vi "Slice Average calc wrapper.vi"(6 "Plot ref":refnum<vi>, 7 "update plot":T2, 10 "HasData?":bool[](array[boolean]), 11 "Plot (unix)":T5[](array[typedef])) -> (3 "Plot (unix)":T5[](array[typedef]), 5 "RightClickCache.slice":T1[](array[typedef]))   [LabVIEW 2021, in "RocketPlot.lvlib"]
uses:
  RocketPlot.lvlib
  TypeDefs/plot datapoint.ctl
  TypeDefs/update plot queue data.ctl
  TypeDefs/RightClickType.ctl
  <vilib>/Utility/miscctls.llb/LVPoint32TypeDef.ctl
  TypeDefs/Slice average.ctl
  b0f39d84-27d9-4b84-b8c3-cf78f35fa78a.vi
  b8f4d68e-665a-4d51-938f-4be5908799fb.vi
  0a7e6c96-3213-4357-8ae2-7647ccf6d38e.vi
  de1cbfd4-f4b0-4655-8da2-e779fdd6673d.vi
  <userlib>/bjustice/Ring Buffer for Time Series Data Strict Accessor/SubVIs/Search for time to keep.vi
  Slice Average calc.vi/aeb3b9b0-3d0b-48fb-8ca9-3c9e8c208765.vi
  Slice Average calc.vi/43998882-4a9d-44ca-a800-b6f182c48d79.vi
  <userlib>/bjustice/Ring Buffer for Time Series Data Strict Accessor/Unix time epoch/Unix_Epoch_in_Labview.vi
  <userlib>/bjustice/Ring Buffer for Time Series Data Strict Accessor/SubVIs/Search for oldest time to keep.vi
  <userlib>/bjustice/Ring Buffer for Time Series Data Strict Accessor/SubVIs/Search for newest time to keep.vi
  <vilib>/Analysis/baseanly.llb/Std Deviation and Variance.vi
  <vilib>/Analysis/8numeric.llb/Uneven Numeric Integration.vi
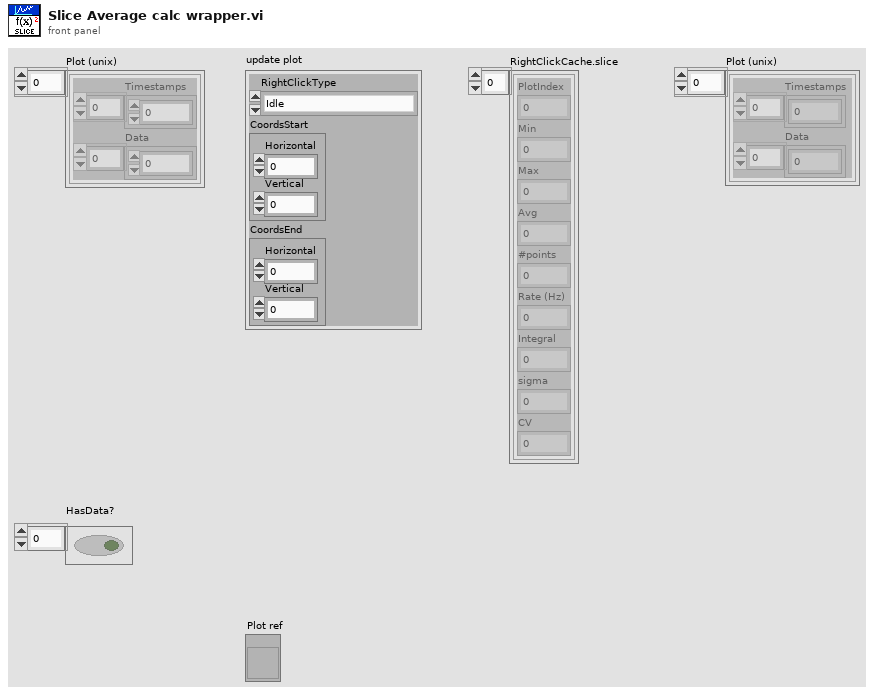
[diagram p1: front panel]
types:
  T1 = typedef "RocketPlot.lvlib/Slice average.ctl" = cluster{"PlotIndex":i32, "Min":dbl, "Max":dbl, "Avg":dbl, "#points":u32, "Rate (Hz)":dbl, "Integral":dbl, "sigma":dbl, "CV":dbl}
  T2 = typedef "RocketPlot.lvlib/update plot queue data.ctl" = cluster{"RightClickType":T3, "CoordsStart":T4, "CoordsEnd":T4}
  T3 = typedef "RocketPlot.lvlib/RightClickType.ctl" = enum16{"Idle", "Delta", "SliceAvg", "Identify"}
  T4 = typedef "LVPoint32TypeDef.ctl" = cluster{"Horizontal":i32, "Vertical":i32}
  T5 = typedef "RocketPlot.lvlib/plot datapoint.ctl" = cluster{"Timestamps":u64[], "Data":dbl[]}
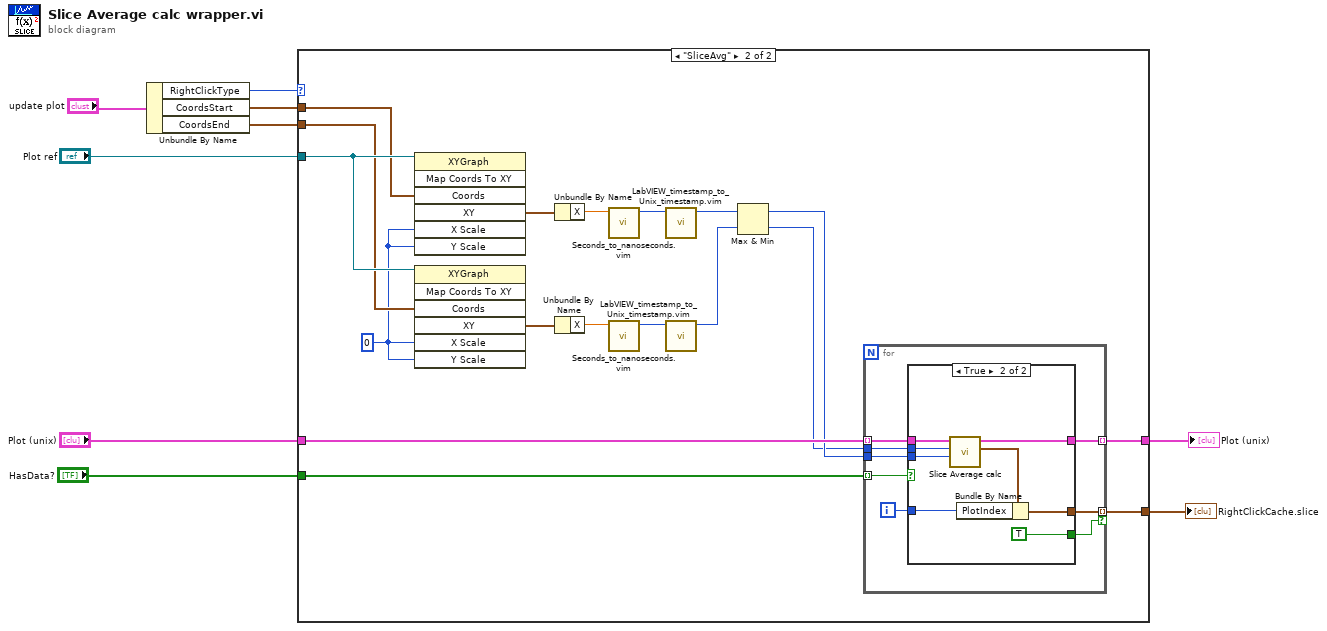
[diagram p0: block diagram]
diagram:
  n1 = Unbundle By Name("update plot") -> ("RightClickType"=w4:T3, "CoordsStart"=w3:T4, "CoordsEnd"=w2:T4)
  n2 = case shown="\"SliceAvg\"" w4 {
    tunnel: "Plot (unix)" -> [w10 w28]
    tunnel: [w10 w27] -> w8
    tunnel: "Plot ref" -> [_ w26]
    tunnel: "HasData?" -> [_ w25]
    tunnel: w3 -> [_ w24]
    tunnel: w2 -> [_ w23]
    tunnel: [_ w22] -> w1
    frame Default {
    }
    frame "SliceAvg" {
      w21 = 0 ("X Scale")
      n3 = invoke class="XYGraph" method="Map Coords To XY"(reference=w26, "Coords"=w24, "X Scale"=w21, "Y Scale"=w21) -> ("XY"=w20:cluster{"X":dbl, "Y":dbl})  [unwired: 3 in, 6 out]
      n4 = invoke class="XYGraph" method="Map Coords To XY"(reference=w26, "Coords"=w23, "X Scale"=w21, "Y Scale"=w21) -> ("XY"=w19:cluster{"X":dbl, "Y":dbl})  [unwired: 3 in, 6 out]
      n5 = Unbundle By Name(w20) -> ("X"=w15:dbl)
      n6 = Unbundle By Name(w19) -> ("X"=w12:dbl)
      n7 = call "Seconds_to_nanoseconds.vim"("timestamp (seconds)"=w15) -> ("timestamp (nanoseconds)"=w16:u64)  [unwired: 10 in]
      n8 = call "Seconds_to_nanoseconds.vim"("timestamp (seconds)"=w12) -> ("timestamp (nanoseconds)"=w13:u64)  [unwired: 10 in]
      n9 = call "LabVIEW_timestamp_to_Unix_timestamp.vim"("LabVIEW timestamp (nanoseconds)"=w16) -> ("Unix timestamp (nanoseconds)"=w14:u64)  [unwired: 10 in]
      n10 = call "LabVIEW_timestamp_to_Unix_timestamp.vim"("LabVIEW timestamp (nanoseconds)"=w13) -> ("Unix timestamp (nanoseconds)"=w11:u64)  [unwired: 10 in]
      n11 = Max & Min(x=w14, y=w11) -> (max(x,y)=w18:u64, min(x,y)=w17:u64)
      n12 = for {
        tunnel: w28 -> [w36] mode=indexing
        tunnel: [w35] -> w27 mode=indexing
        tunnel: [w34] -> w22 mode=indexing if=w29
        tunnel: w17 -> [w33]
        tunnel: w18 -> [w32]
        tunnel: w25 -> [w31] mode=indexing
        i -> [w30]
        n13 = case shown="True" w31 {
          tunnel: w36 -> [w37 w45]
          tunnel: [w37 w44] -> w35
          tunnel: [_ w39] -> w34
          tunnel: w33 -> [_ w43]
          tunnel: w32 -> [_ w42]
          tunnel: w30 -> [_ w40]
          tunnel: [_ TRUE] -> w29
          frame False {
          }
          frame True {
            n14 = call "Slice Average calc.vi"("end time (unix,ns)"=w42, "start time (unix,ns)"=w43, "Plot (unix)"=w45) -> ("slice average"=w41:T1, "Plot (unix)"=w44:T5)  [unwired: 7 in]
            n15 = Bundle By Name(cluster=w41, "PlotIndex"=w40) -> (w39:T1)
          }
        }
      }
    }
  }
  "Plot (unix)" <- w8
  "RightClickCache.slice" <- w1
